vi "Write Serial Number.vi"(6 "error in":errorcluster, 7 "Serial number":u32, 8 "MaxRead":i32, 9 "Channel in":u16) -> (0 "error out":errorcluster, 1 "Messages":T1(array[cluster]), 2 "Pass":bool, 3 "Channel out":u16)   [LabVIEW 2023]
uses:
  4f930f32-d09a-43ef-bca1-8b214b378bd5.vi
  Communication/PCAN2023/PCAN API.lvlib
  f2a2f8e7-f6f6-4780-9dbf-cb0b851d76e9.vi
  536f1125-b32c-464d-83f3-71b6f093e3b0.vi
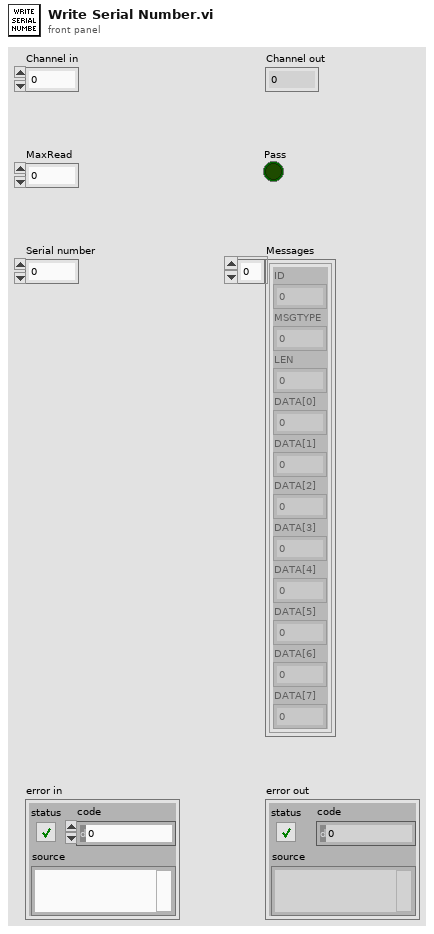
[diagram p1: front panel]
types:
  T1 = cluster{"ID":u32, "MSGTYPE":u8, "LEN":u8, "DATA[0]":u8, "DATA[1]":u8, "DATA[2]":u8, "DATA[3]":u8, "DATA[4]":u8, "DATA[5]":u8, "DATA[6]":u8, "DATA[7]":u8}[]
  T2 = cluster{"ID":u32, "MSGTYPE":u8, "LEN":u8, "DATA[0]":u8, "DATA[1]":u8, "DATA[2]":u8, "DATA[3]":u8, "DATA[4]":u8, "DATA[5]":u8, "DATA[6]":u8, "DATA[7]":u8}
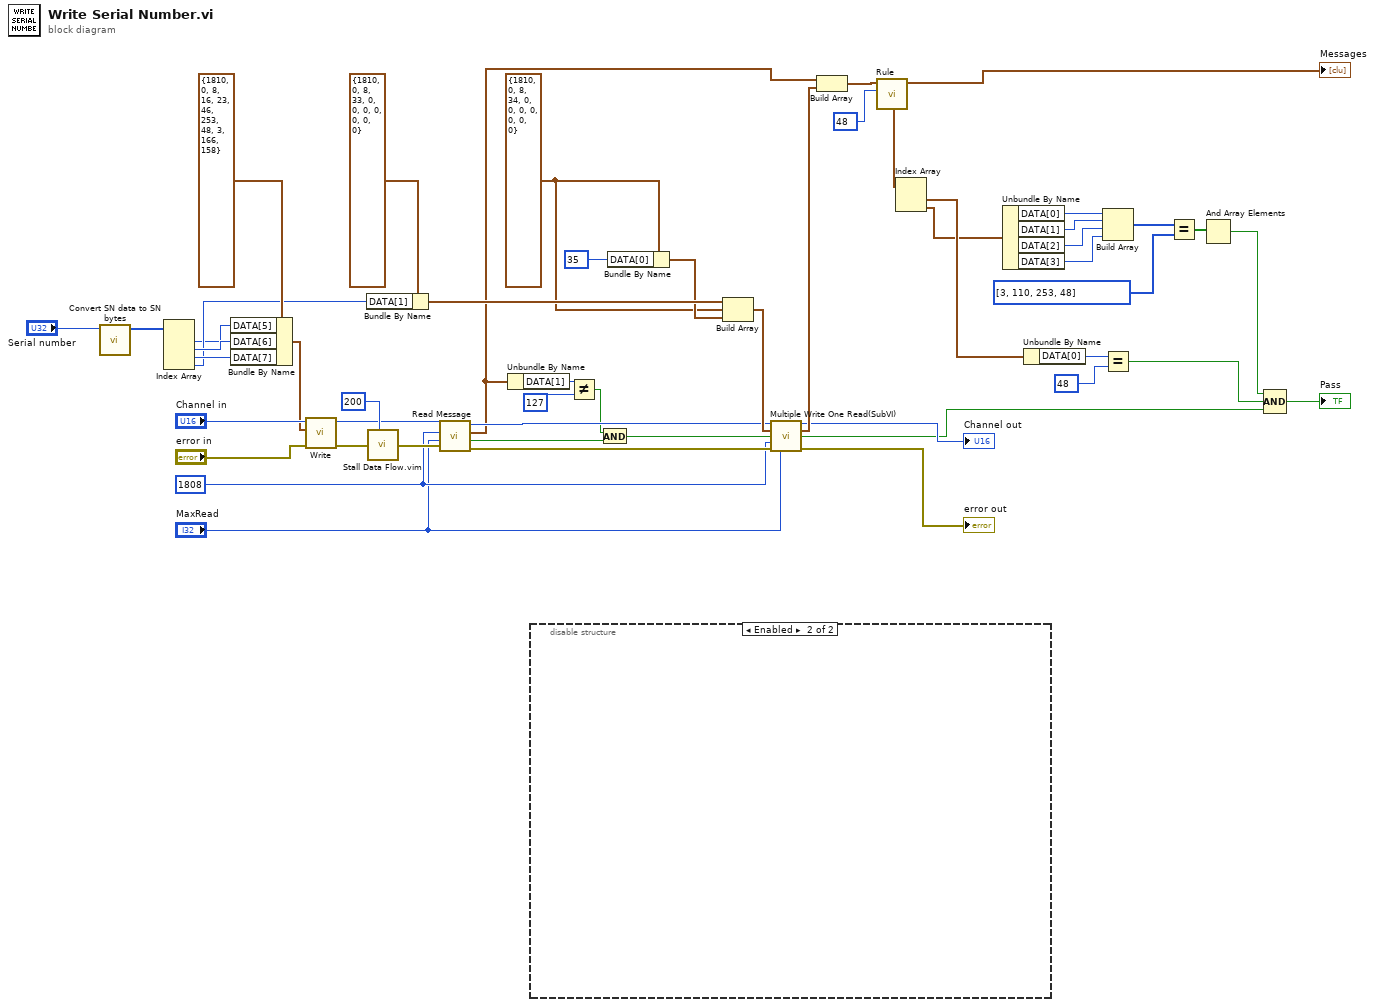
[diagram p0: block diagram]
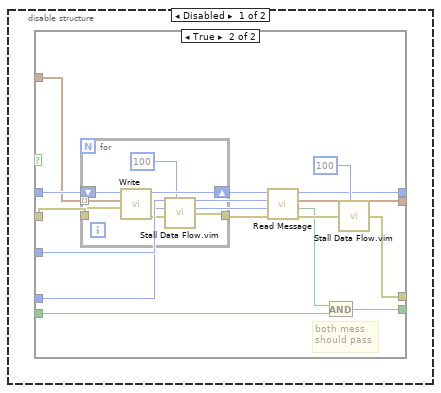
[diagram p2: hidden frame]
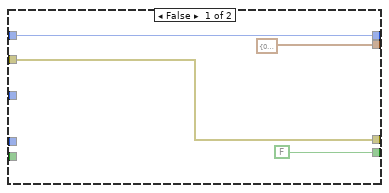
[diagram p3: hidden frame]
diagram:
  w34 = T2 {"ID"=1810, "MSGTYPE"=0, "LEN"=8, "DATA[0]"=34, "DATA[1]"=0, "DATA[2]"=0, "DATA[3]"=0, "DATA[4]"=0, "DATA[5]"=0, "DATA[6]"=0, "DATA[7]"=0} ("MessageBuffer")
  (unwired) u32 200 ("milliseconds to wait")
  w14 = u32 1808 ("ID")
  n1 = call "Convert SN data to SN bytes.vi"("SN"="Serial number") -> ("SN Data Bytes"=w30:u8[])  [unwired: 10 in]
  n2 = Index Array(array=w30) -> (element #1=w32:u8, element #2=w42:u8, element #3=w41:u8, element #4=w39:u8)  [unwired: 4 in]
  n3 = Bundle By Name(cluster=T2 {"ID"=1810, "MSGTYPE"=0, "LEN"=8, "DATA[0]"=16, "DATA[1]"=23, "DATA[2]"=46, "DATA[3]"=253, "DATA[4]"=48, "DATA[5]"=3, "DATA[6]"=166, "DATA[7]"=158} ("MessageBuffer"), "DATA[5]"=w32, "DATA[6]"=w42, "DATA[7]"=w41) -> (w38:T2)
  n4 = call "Write.vi"("error in"="error in", "MessageBuffer"=w38, "Channel"="Channel in") -> ("error out"=w47:errorcluster, "Channel out"=w18:u16)  [unwired: 5 in, 2 out]
  n5 = Bundle By Name(cluster=T2 {"ID"=1810, "MSGTYPE"=0, "LEN"=8, "DATA[0]"=33, "DATA[1]"=0, "DATA[2]"=0, "DATA[3]"=0, "DATA[4]"=0, "DATA[5]"=0, "DATA[6]"=0, "DATA[7]"=0} ("MessageBuffer"), "DATA[1]"=w39) -> (w36:T2)
  n6 = call "Stall Data Flow.vim"("value in"=w47, "milliseconds to wait"=u32 200) -> ("value out"=w17:errorcluster)  [unwired: 1 out]
  n7 = call "Read Message.vi"("error in"=w17, "MaxRead"="MaxRead", "ID"=w14, "Channel in"=w18) -> ("error out"=w15:errorcluster, "Passed"=w11:bool, "Last Message"=w5:T2, "Channel out"=w16:u16)  [unwired: 3 in, 1 out]
  n8 = Unbundle By Name(w5) -> ("DATA[1]"=w45:u8)
  n9 = disable-structure shown="Enabled" {
    frame Disabled {
      n10 = case shown="True" {
        selector: _ -> [_ _]
        tunnel: _ -> [w54 w70]
        tunnel: _ -> [w52 w69]
        tunnel: [w52 w68] -> _
        tunnel: [FALSE w64] -> _
        tunnel: [w54 w61] -> _
        tunnel: _ -> [_ w67]
        tunnel: [T2 {"ID"=0, "MSGTYPE"=0, "LEN"=0, "DATA[0]"=0, "DATA[1]"=0, "DATA[2]"=0, "DATA[3]"=0, "DATA[4]"=0, "DATA[5]"=0, "DATA[6]"=0, "DATA[7]"=0} w56] -> _
        tunnel: _ -> [_ w65]
        tunnel: _ -> [_ w59]
        tunnel: _ -> [_ w58]
        frame False {
        }
        frame True {
          # "both mess\nshould pass"
          n11 = for {
            tunnel: w67 -> [w73] mode=indexing
            shift-right: [w75] -> w63
            shift-left: w70 -> [w77]
            tunnel: w69 -> [w76]
            tunnel: [w74] -> w62
            n12 = call "Write.vi"("error in"=w76, "MessageBuffer"=w73, "Channel"=w77) -> ("error out"=w71:errorcluster, "Channel out"=w75:u16)  [unwired: 5 in, 2 out]
            n13 = call "Stall Data Flow.vim"("value in"=w71, "milliseconds to wait"=u32 100) -> ("value out"=w74:errorcluster)  [unwired: 1 out]
          }
          n14 = call "Read Message.vi"("error in"=w62, "MaxRead"=w58, "ID"=w59, "Channel in"=w63) -> ("error out"=w60:errorcluster, "Passed"=w57:bool, "Last Message"=w56:T2, "Channel out"=w61:u16)  [unwired: 3 in, 1 out]
          n15 = And(x=w57, y=w65) -> (x .and. y?=w64:bool)
          n16 = call "Stall Data Flow.vim"("value in"=w60, "milliseconds to wait"=u32 100) -> ("value out"=w68:errorcluster)  [unwired: 1 out]
        }
      }
    }
    frame Enabled {
    }
  }
  n17 = Not Equal?(x=w45, y=u8 127) -> (x != y?=w12:bool)
  n18 = And(x=w12, y=w11) -> (x .and. y?=w10:bool)
  n19 = Bundle By Name(cluster=w34, "DATA[0]"=u8 35) -> (w35:T2)
  n20 = Build Array(w36, w34, w35) -> (w33:T1)
  n21 = call "Multiple Write One Read(SubVI).vi"("Channel in"=w16, "Messages to write"=w33, "Mess 1 Passed"=w10, "ID"=w14, "error in"=w15, "MaxRead"="MaxRead") -> ("Channel out"=→"Channel out":u16, "Last Message"=w9:T2, "Messages passed"=w7:bool, "error out"=→"error out":errorcluster)  [unwired: 6 in]
  n22 = Build Array(w5, w9) -> (w6:T1)
  n23 = call "Rule.vi"("Case"=u8 48 ("y"), "Array in"=w6) -> ("Array out"=w4:T1)  [unwired: 9 in]
  "Messages" <- w4
  n24 = Index Array(array=w4) -> (element #1=w3:T2, element #2=w2:T2)  [unwired: 2 in]
  n25 = Unbundle By Name(w2) -> ("DATA[0]"=w26:u8, "DATA[1]"=w25:u8, "DATA[2]"=w24:u8, "DATA[3]"=w23:u8)
  n26 = Unbundle By Name(w3) -> ("DATA[0]"=w27:u8)
  n27 = Build Array(w26, w25, w24, w23) -> (w22:u8[])
  n28 = Equal?(x=w27, y=u8 48) -> (x = y?=w29:bool)
  n29 = Equal?(x=w22, y=u8[] [3, 110, 253, 48]) -> (x = y?=w20:bool[])
  n30 = And Array Elements(Boolean array=w20) -> (logical AND=w19:bool)
  n31 = Compound Arithmetic op=AND(w19, w29, w7) -> (→"Pass":bool)
